vi "Read Module Name.vi"(8 "error in (no error)":errorcluster, 11 "RemIO Module in":refnum<class "RemIO Module.lvclass">) -> (0 "error out":errorcluster, 2 "Module Name":string, 3 "RemIO Module out":refnum<class "RemIO Module.lvclass">)   [LabVIEW 2019, in "Modules.lvlib" / "RemIO Module.lvclass"]
uses:
  RemIO Module.lvclass
  RemIO Module.lvclass/RemIO Module.ctl
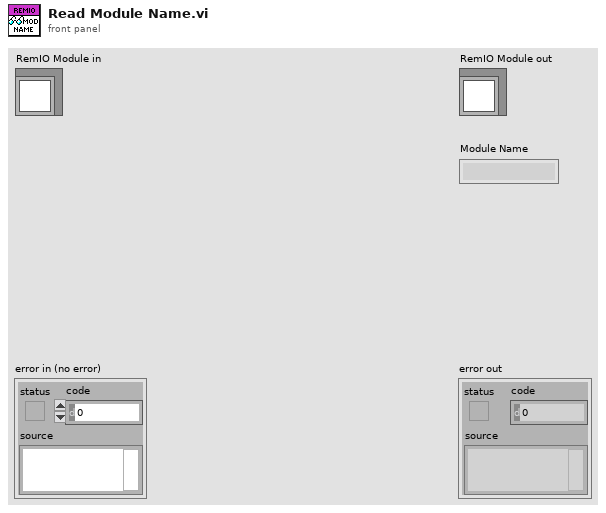
[diagram p1: front panel]
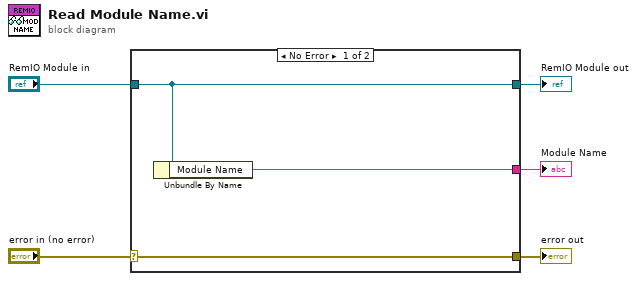
[diagram p0: block diagram]
diagram:
  n1 = case shown="No Error" "error in (no error)" {
    selector: "error in (no error)" -> [w8 w9]
    tunnel: [w8 w9] -> w4
    tunnel: [w7 w10] -> w2
    tunnel: "RemIO Module in" -> [w7 w10]
    tunnel: [w6 _] -> w1
    frame No Error {
      n2 = Unbundle By Name(w7) -> ("Module Name"=w6:string)
    }
    frame Error {
    }
  }
  "error out" <- w4
  "RemIO Module out" <- w2
  "Module Name" <- w1
